vi "Create Event References and Registrations.vi"(8 "error in (no error)":errorcluster) -> (0 "error out":errorcluster, 3 "Event-References":T1)   [LabVIEW 2018, in "Actor.lvclass"]
uses:
  Actor.lvclass
  Event-References.ctl
  Stop.ctl
  Actor Class Launched.ctl
  Example-Request.ctl
  Example-Reply.ctl
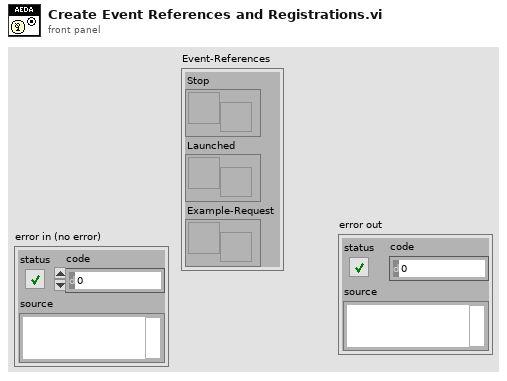
[diagram p1: front panel]
types:
  T1 = typedef "Actor.lvclass/Event-References.ctl" = cluster{"Stop":refnum<user-event>, "Launched":refnum<user-event>, "Example-Request":refnum<user-event>}
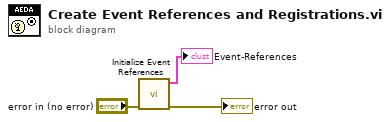
[diagram p0: block diagram]
diagram:
  n1 = call "Initialize Event References.vi"("error in (no error)"="error in (no error)") -> ("error out"=→"error out":errorcluster, "Event-References"=→"Event-References":T1)  [unwired: 9 in]
